vi "Send Register AEs.vi"(7 "Message Priority (Normal)":T2=enum."Normal", 8 "error in (no error)":errorcluster, 10 "Register Info":T1, 11 "Message Enqueuer":refnum<class "Message Enqueuer.lvclass">) -> (0 "error out":errorcluster, 3 "Message Enqueuer out":refnum<class "Message Enqueuer.lvclass">)   [LabVIEW 2015, in "CS++PVMonitor.lvlib" / "Register AEs Msg.lvclass"]
doc: "Sends the <B>CS++PVMonitor.lvlib:Register AEs Msg.lvclass</B> message.\n\n<B>CS++PVMonitor.lvlib:CS++PVMonitor.lvclass:Register AEs.vi</B> Description:\n\nRegister alarm and event monitoring for process variables."
uses:
  Register AEs Msg.lvclass
  <vilib>/ActorFramework/Message Enqueuer/Message Enqueuer.lvclass
  <vilib>/ActorFramework/Message Enqueuer/Message Priority.ctl
  CS++AEUpdate Msg/CS++AEUpdate Msg.lvclass
  Register AEs Msg.lvclass/Register AEs Msg.ctl
  <vilib>/ActorFramework/Message Enqueuer/Message Enqueuer.lvclass/Message Enqueuer.ctl
  <vilib>/ActorFramework/Message Priority Queue/Priority Enqueue.vi
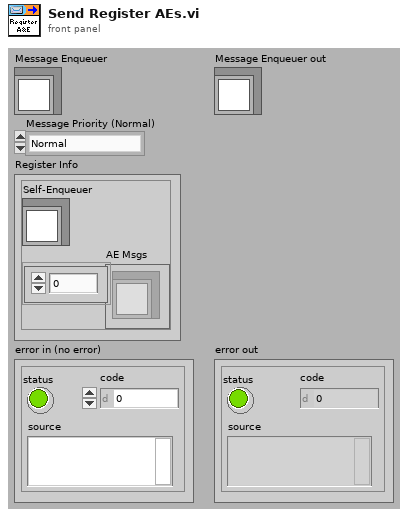
[diagram p1: front panel]
types:
  T1 = cluster{"Self-Enqueuer":refnum<class "Message Enqueuer.lvclass">, "AE Msgs":refnum<class "CS++AEUpdate Msg.lvclass">[]}
  T2 = typedef "Actor Framework.lvlib/Message Enqueuer.lvclass/Message Priority.ctl" = enum16{"Low", "Normal", "High"}
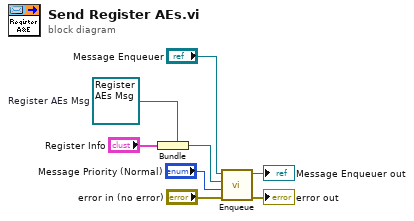
[diagram p0: block diagram]
diagram:
  w2 = refnum<class "Register AEs Msg.lvclass"> refnum  # Register AEs Msg
  n1 = Bundle(cluster=w2, "Register Info") -> (w5:refnum<class "Register AEs Msg.lvclass">)
  n2 = call <vilib>:"Enqueue.vi"("error in (no error)"="error in (no error)", "Message Priority (Normal)"="Message Priority (Normal)", "Message"=w5, "Message Enqueuer in"="Message Enqueuer") -> ("error out"=→"error out":errorcluster, "Message Enqueuer out"=→"Message Enqueuer out":refnum<class "Message Enqueuer.lvclass">)  [unwired: 6 in]
